vi "HALF-IMS control.vi"() -> ()   [LabVIEW 2017]
uses:
  <vilib>/Utility/error.llb/DialogType.ctl
  <vilib>/Utility/file.llb/Read Delimited Spreadsheet (DBL).vi
panel:
  in  "Stop 2":bool
  out "Read Sample rate (act.)":dbl
  in  "Leads \nCurrent only/Voltage audit + current":bool
  out "Generated Sample rate (act.)":dbl
  in  "Plot Display? \nOff/On":bool
  in  "sweep or Airflow control":bool
  out "Current or last file saved:":string
  in  "Run number":dbl
  in  "file path (dialog if empty)":path=path "C:/Users/bioMEMS/Desktop/Yuriy/Data/W16/031716 dev727 UV sweeps/inputs@10.csv"
  in  "Device":string
  in  "Test run or Use Filename":bool
  in  "Voltage":string
  in  "output frequency":string
  in  "airflow":string
  in  "Chemical name":string
  out "Airflow readings":string
  in  "Vacuum":dbl
  in  "Dilution":dbl
  in  "M Sal":dbl
  in  "Nitrogen":dbl
  out "Monitor Output Voltages":cluster{dbl, dbl, dbl, dbl}(graph)
  in  "Turn on Airflow control?":bool
  in  "VL":dbl
  in  "VS":dbl
  in  "Stop":bool
  out "Loop finished?":bool
  in  "Voltage control inputs: file or custom inputs":bool
  out "+ bias (-ions)":dbl(graph)
  out "- bias (+ions)":dbl(graph)
  in  "Output points (use same as rate or lower)":i32=1000
  in  "Voltage Output rate (Hz)":dbl=1000.0
  in  "Sample Rate (Hz)":dbl=1000.0
  in  "Number of Samples\n(use same as rate or lower)":i32=100
  # "© The Regents of the University of California, Davis campus, 2019. This material is available as open source for research and personal use under a Creative Commons Attribution-NonCommercial-NoDerivatives 4.0 International Public License (https://creativecommons.org/licenses/by-nc-nd/4.0/)."
  # "Airflow Control"
  # "Filename"
  # "MUST BE SPECIFIED\neven if not in use"
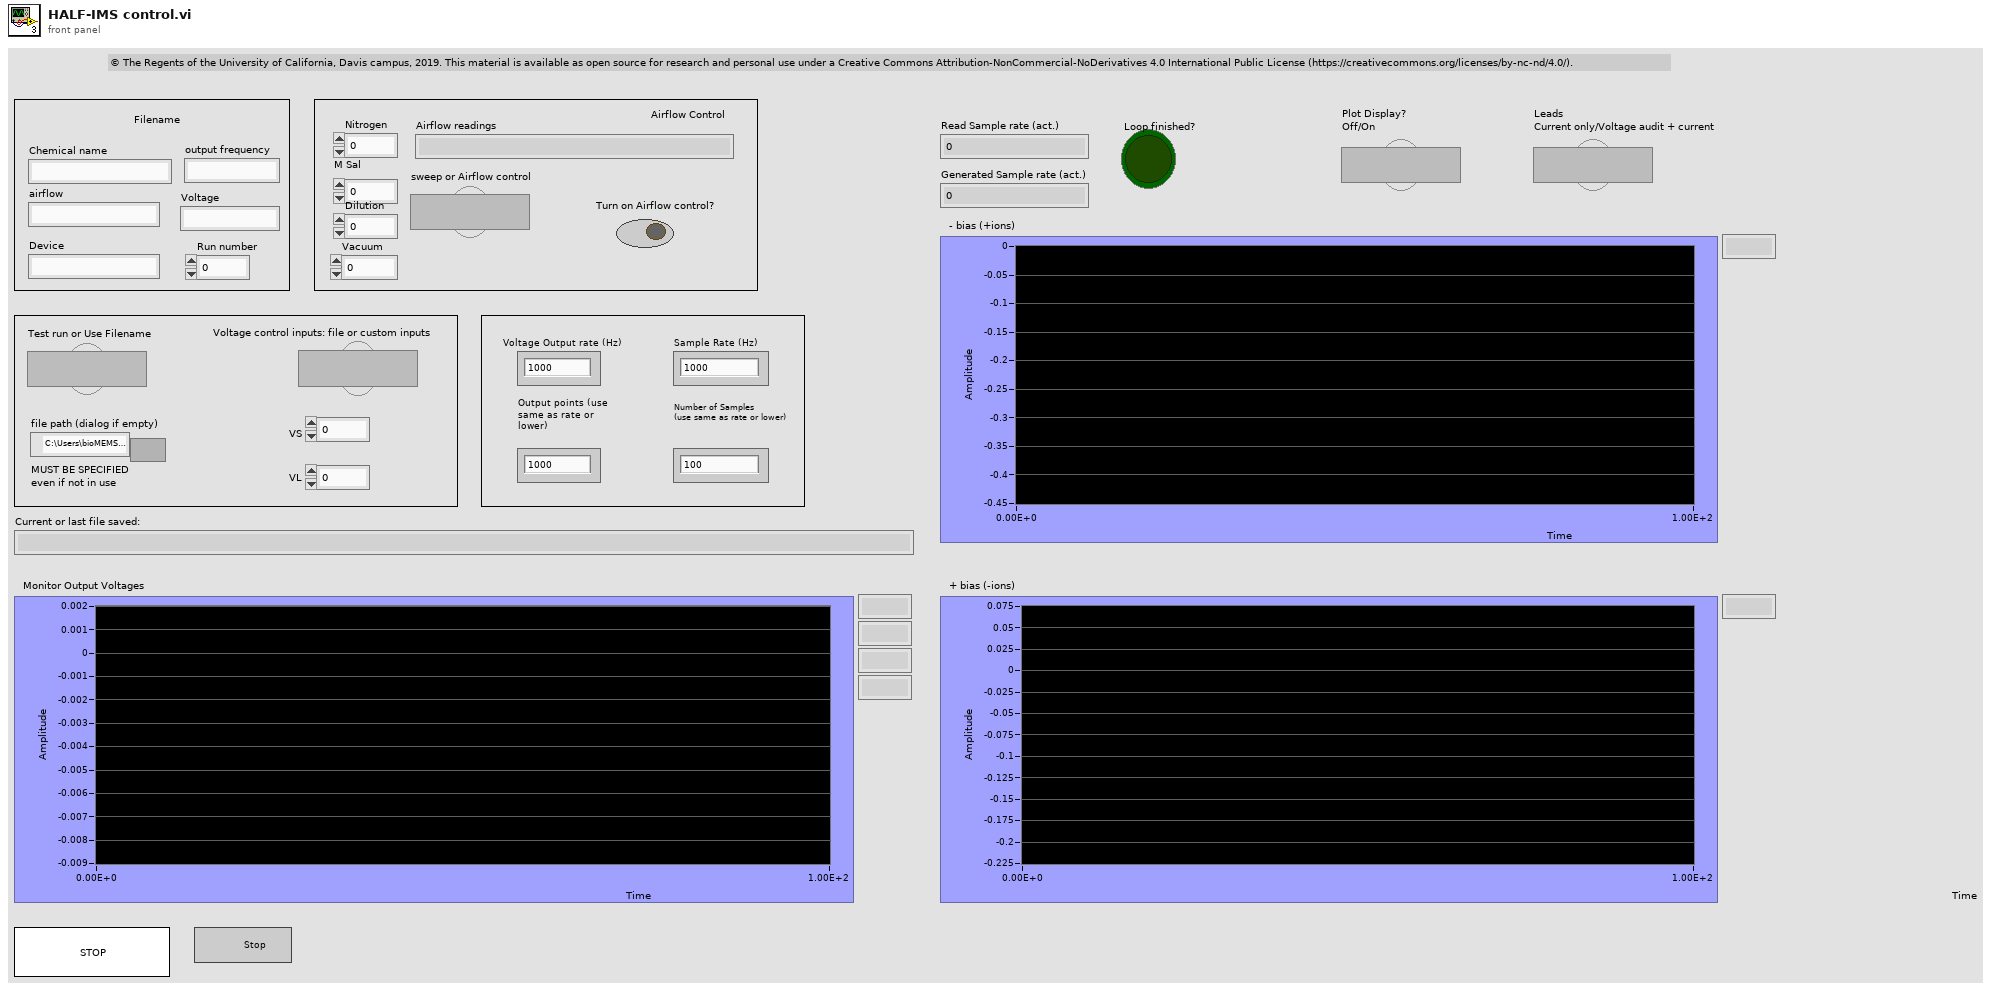
[diagram p1: front panel]
types:
  T1 = enum16{"open", "replace", "create", "open or create", "replace or create", "replace or create with confirmation"}
  T2 = typedef "DialogType.ctl" = u16
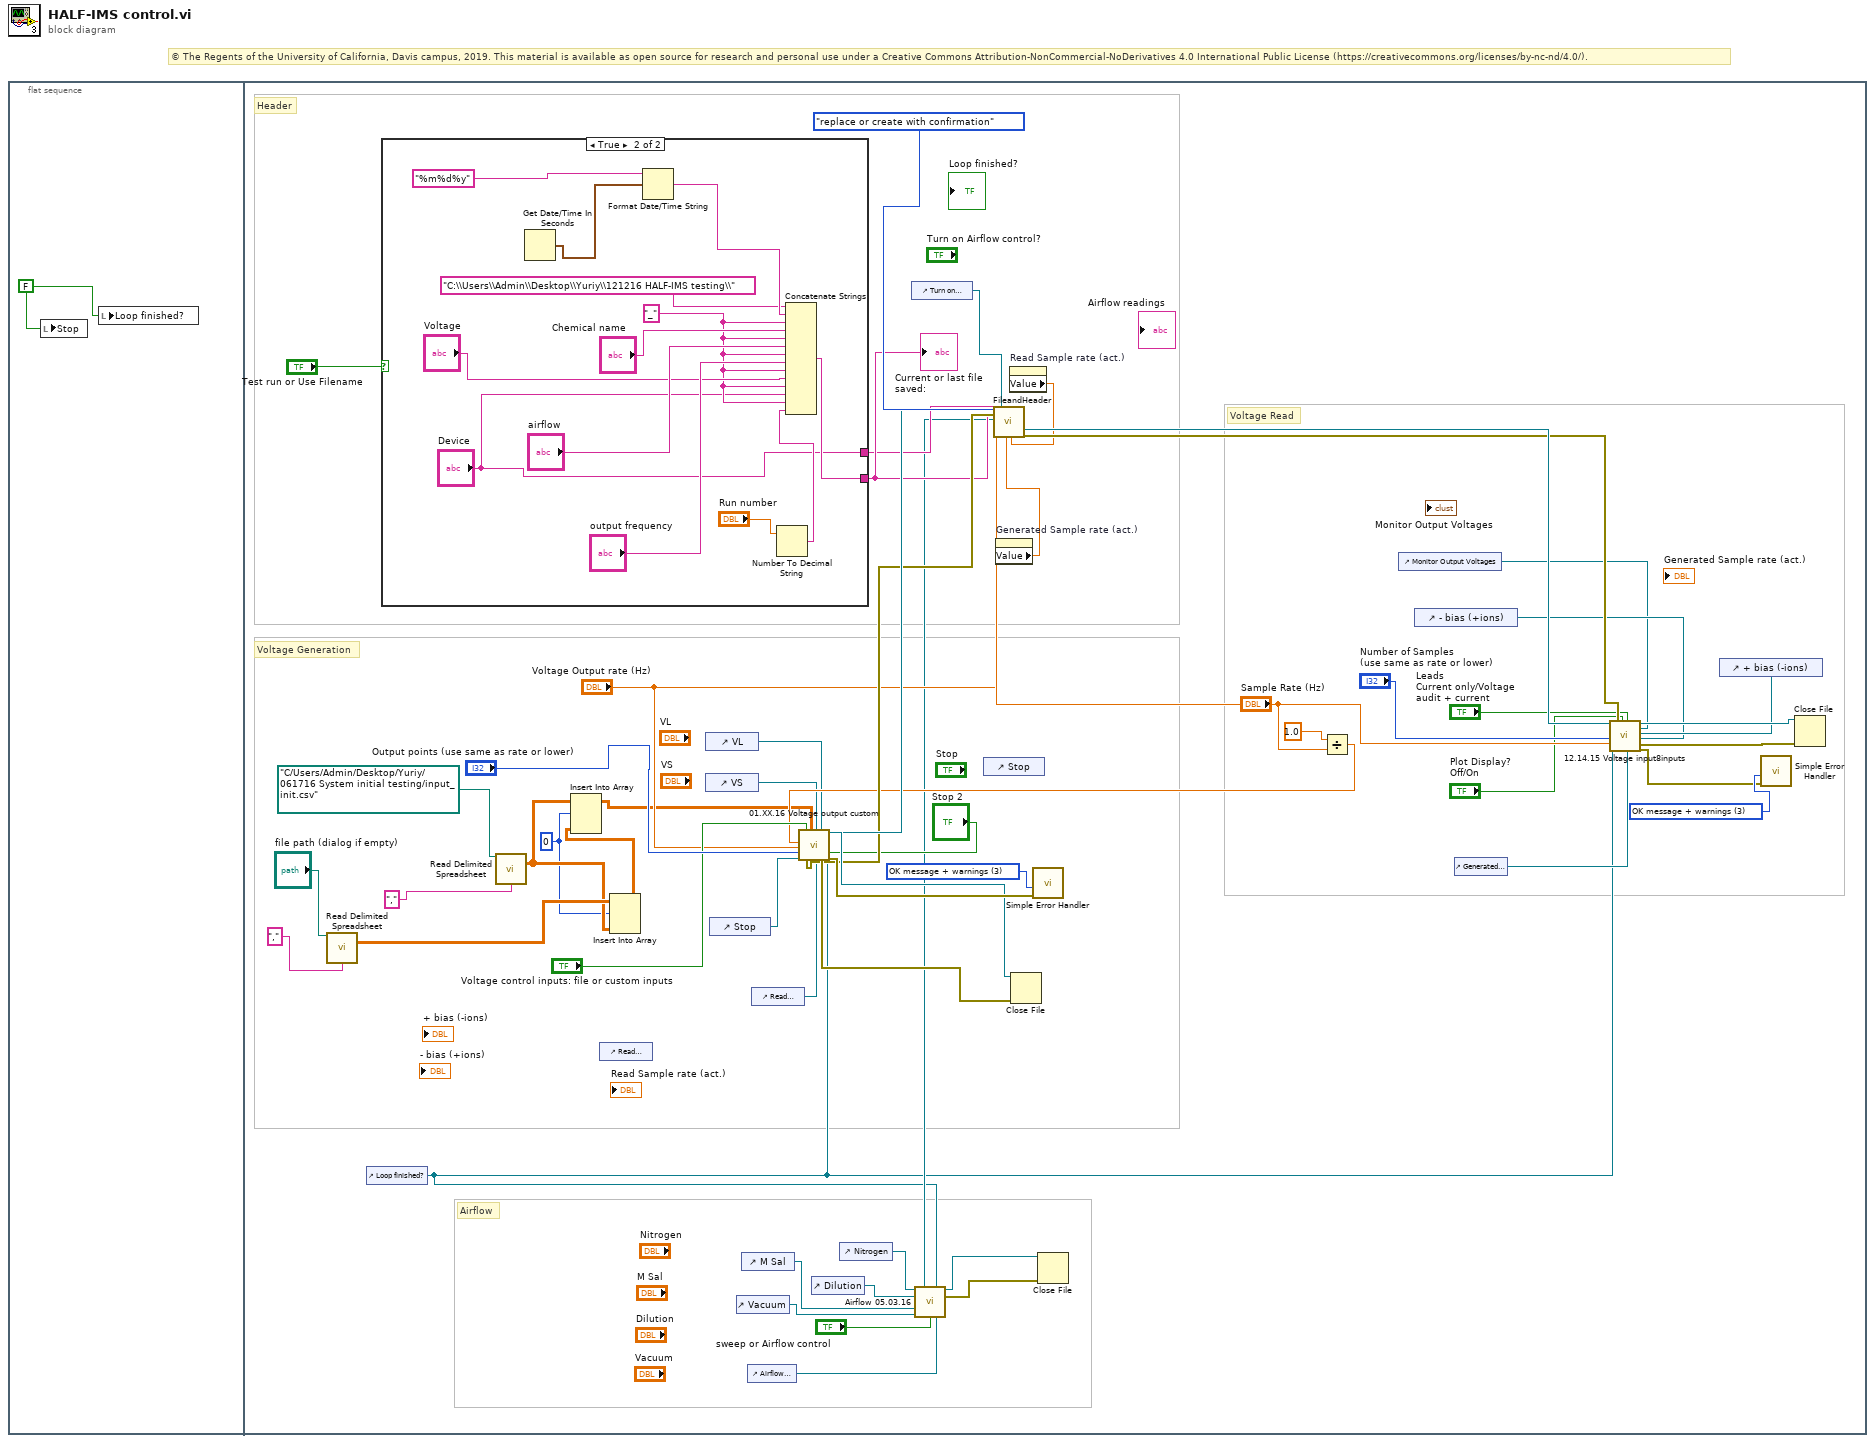
[diagram p0: block diagram]
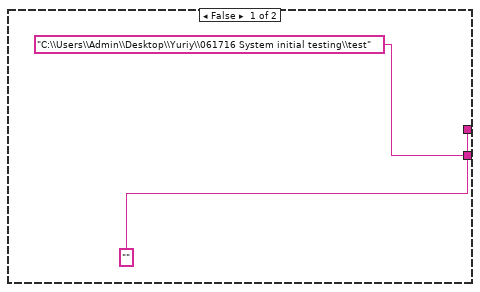
[diagram p2: hidden frame]
diagram:
  # "© The Regents of the University of California, Davis campus, 2019. This material is available as open source for research and personal use under a Creative Commons Attribution-NonCommercial-NoDerivatives 4.0 International Public License (https://creativecommons.org/licenses/by-nc-nd/4.0/)."
  n1 = flat-sequence {
    frame #0 {
      w1 = FALSE ("logical OR")
      n2 = local write "Stop"(w1) -> ()
      n3 = local write "Loop finished?"(w1) -> ()
    }
    frame #1 {
      w2 = 0 ("index (row)")
      w55 = T2 3 items=["no dialog", "OK message", "continue or stop message", "OK message + warnings", "continue/stop + warnings"] ("type of dialog (OK msg:1)")
      w56 = T2 3 items=["no dialog", "OK message", "continue or stop message", "OK message + warnings", "continue/stop + warnings"] ("type of dialog (OK msg:1)")
      # "Airflow"
      # "Voltage Generation"
      # "Voltage Read"
      # "Header"
      n4 = call-poly <vilib>:"Read Delimited Spreadsheet.vi"("file path (dialog if empty)"="file path (dialog if empty)", "delimiter (\\t)"="," ("delimiter (\\t)")) -> ("all rows"=w26:dbl[][])  [unwired: 8 in, 5 out]
      n5 = control-ref of="Loop finished?"() -> (w10:refnum<vi>)
      n6 = case shown="True" "Test run or Use Filename" {
        tunnel: ["C:\\Users\\Admin\\Desktop\\Yuriy\\061716 System initial testing\\test" ("string") w65] -> w30
        tunnel: ["" ("Device") "Device"] -> w16
        frame False {
        }
        frame True {
          w63 = "_" ("string")
          n7 = Get Date/Time In Seconds() -> (seconds since 1Jan1904=w67:timestamp)
          n8 = Format Date/Time String(time format string (%c)="%m%d%y", seconds (now)=w67) -> (date/time string=w68:string)  [unwired: 1 in]
          n9 = Number To Decimal String(number="Run number") -> (decimal integer string=w61:string)  [unwired: 1 in]
          n10 = Concatenate Strings("C:\\Users\\Admin\\Desktop\\Yuriy\\121216 HALF-IMS testing\\" ("string"), w68, w63, "Chemical name", w63, "airflow", w63, "output frequency", w63, "Voltage", w63, "Device", w63, w61) -> (w65:string)
        }
      }
      "Current or last file saved:" <- w30
      n11 = call-poly <vilib>:"Read Delimited Spreadsheet.vi"("file path (dialog if empty)"=path "C:/Users/Admin/Desktop/Yuriy/061716 System initial testing/input_init.csv", "delimiter (\\t)"="," ("delimiter (\\t)")) -> ("all rows"=w5:dbl[][])  [unwired: 8 in, 5 out]
      n12 = control-ref of="Read Sample rate (act.)"() -> ()  [unwired: 1 out]
      n13 = Insert Into Array(array=w26, index (row)=w2, new element=w5) -> (w4:dbl[][])  [unwired: 1 in]
      n14 = Insert Into Array(array=w5, index (row)=w2, new element=w4) -> (w3:dbl[][])  [unwired: 1 in]
      n15 = control-ref of="VL"() -> (w34:refnum<vi>)
      n16 = control-ref of="VS"() -> (w35:refnum<vi>)
      n17 = control-ref of="Stop"() -> (w40:refnum<vi>)
      n18 = control-ref of="Vacuum"() -> (w12:refnum<vi>)
      n19 = control-ref of="M Sal"() -> (w13:refnum<vi>)
      n20 = control-ref of="Airflow readings"() -> (w6:refnum<vi>)
      n21 = control-ref of="Read Sample rate (act.)"() -> (w20:refnum<vi>)
      n22 = control-ref of="Dilution"() -> (w15:refnum<vi>)
      n23 = control-ref of="Nitrogen"() -> (w14:refnum<vi>)
      n24 = control-ref of="Turn on Airflow control?"() -> (w33:refnum<vi>)
      n25 = control-ref of="Stop"() -> ()  [unwired: 1 out]
      n26 = property on="Generated Sample rate (act.)" class="DigNum (strict)"() -> ("Value"=w18:dbl)  [unwired: 2 in, 2 out]
      n27 = property on="Read Sample rate (act.)" class="DigNum (strict)"() -> ("Value"=w17:dbl)  [unwired: 2 in, 2 out]
      n28 = call "FileandHeader.vi"("operation (0:open)"=T1."replace or create with confirmation", "string"=w30, "Specified sampling rate"="Sample Rate (Hz)", "Specified generated frequency (Hz)"="Voltage Output rate (Hz)", "reference"=w33, "Device name"=w16, "Gen sample rate"=w18, "Read sample rate"=w17) -> ("write"=w46:refnum<file>, "error out 2"=w45:errorcluster, "airflow refnum out"=w11:refnum<file>, "read"=w44:refnum<file>, "error out"=w43:errorcluster)  [unwired: 6 in, 1 out]
      n29 = call "Airflow 05.03.16.vi"("Helium"=w14, "Write refnum In"=w11, "Stop in"=w10, "Nitrogen"=w15, "Chemical"=w13, "Vacuum"=w12, "Boolean"="sweep or Airflow control", "String out"=w6) -> ("refnum out 2"=w9:refnum<file>, "error out"=w7:errorcluster)  [unwired: 4 in, 2 out]
      n30 = Close File(refnum=w9, error in=w7) -> ()  [unwired: 2 out]
      n31 = Divide(x=1.0 ("y"), y="Sample Rate (Hz)") -> (x/y=w37:dbl)
      n32 = call "01.XX.16 Voltage output custom.vi"("Write refnum in"=w46, "Step time"=w37, "Sample Rate"="Voltage Output rate (Hz)", "Number of Samples"="Output points (use same as rate or lower)", "Stop Custom In"=w40, "Custom or file"="Voltage control inputs: file or custom inputs", "error in 2"=w45, "array 2"=w3, "VS in"=w35, "Sample Rate (actual)"=w20, "VL in"=w34, "Loop done logical"=w10, "Stop"="Stop 2") -> ("error out 2"=w49:errorcluster, "Write refnum out"=w48:refnum<file>, "error out"=w54:errorcluster)  [unwired: 4 in]
      n33 = Close File(refnum=w48, error in=w49) -> ()  [unwired: 2 out]
      n34 = call <vilib>:"Simple Error Handler.vi"("type of dialog (OK msg:1)"=w56, "error in (no error)"=w54) -> ()  [unwired: 3 in, 5 out]
      n35 = control-ref of="Monitor Output Voltages"() -> (w32:refnum<vi>)
      n36 = control-ref of="- bias (+ions)"() -> (w36:refnum<vi>)
      n37 = control-ref of="Generated Sample rate (act.)"() -> (w22:refnum<vi>)
      n38 = control-ref of="+ bias (-ions)"() -> (w41:refnum<vi>)
      n39 = call "12.14.15 Voltage input8inputs.vi"("refnum Write file in"=w44, "Stop in"=w10, "Number of Samples"="Number of Samples\n(use same as rate or lower)", "Sample Rate"="Sample Rate (Hz)", "error in 2"=w43, "Display? \nOff/On"="Plot Display? \nOff/On", "Boolean"="Leads \nCurrent only/Voltage audit + current", "Sample rate (actual)"=w22, "Plot Output"=w32, "Plot 1 ref"=w41, "Plot 2 ref"=w36) -> ("error out 2"=w50:errorcluster, "refnum Write file out"=w51:refnum<file>, "error out"=w52:errorcluster)  [unwired: 6 in]
      n40 = call <vilib>:"Simple Error Handler.vi"("type of dialog (OK msg:1)"=w55, "error in (no error)"=w52) -> ()  [unwired: 3 in, 5 out]
      n41 = Close File(refnum=w51, error in=w50) -> ()  [unwired: 2 out]
    }
  }
